vi "HTTP Error.vi"(1 "Error code options":T3={"1xx (info)"=FALSE, "2xx (success)"=FALSE, "3xx (redirect)"=FALSE, "4xx (client error)"=TRUE, "5xx (server error)"=TRUE, "Other"=TRUE}, 5 "Header":string="HTTP/1.1 301 Moved Permanently\r\nLocation: http://www.google.com/\r\nContent-Type: text/html; charset=UTF-8\r\nDate: Thu, 22 Mar 2012 21:41:48 GMT\r\nExpires: Sat, 21 Apr 2012 21:41:48 GMT\r\nCache-Control: public, max-age=2592000\r\nServer: gws\r\nContent-Length: 219\r\nX-XSS-Protection: 1; mode=block\r\nX-Frame-Options: SAMEORIGIN", 7 "body":string, 11 "error in (no error)":errorcluster) -> (4 "HTTP response code":T2, 6 "Header (dup)":string="HTTP/1.1 301 Moved Permanently\r\nLocation: http://www.google.com/\r\nContent-Type: text/html; charset=UTF-8\r\nDate: Thu, 22 Mar 2012 21:41:48 GMT\r\nExpires: Sat, 21 Apr 2012 21:41:48 GMT\r\nCache-Control: public, max-age=2592000\r\nServer: gws\r\nContent-Length: 219\r\nX-XSS-Protection: 1; mode=block\r\nX-Frame-Options: SAMEORIGIN", 8 "body (dup)":string, 10 "Header Values":T1[](array[typedef]), 14 "Error log":string, 15 "error out":errorcluster)   [LabVIEW 2020, in "Blue Easy HTTP OpenSource.lvlib"]
doc: "Turns HTTP Response Codes into the proper warning or error.\n\nHTTP 1xx Informational - Warning\nHTTP 2xx Successful - Warning\nHTTP 3xx Redirection - Error\nHTTP 4xx Client Error - Error\nHTTP 5xx Server Error - Error"
uses:
  Blue Easy HTTP OpenSource.lvlib
  HTTP error on codes.ctl
  HTTP response code.ctl
  HTTP Header.ctl
  <vilib>/dlg_ctls.llb/Space Constant.vi
  <vilib>/Utility/error.llb/Trim Whitespace.vi
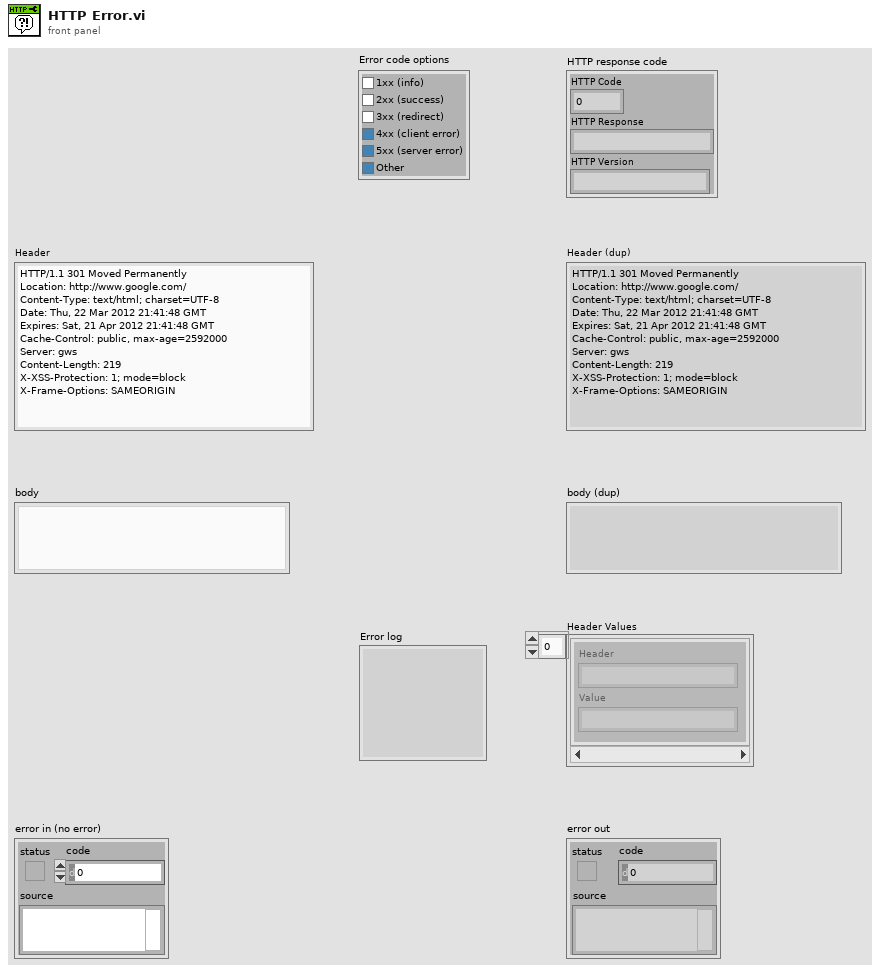
[diagram p1: front panel]
types:
  T1 = typedef "Blue Easy HTTP OpenSource.lvlib/HTTP Header.ctl" = cluster{"Header":string, "Value":string}
  T2 = typedef "Blue Easy HTTP OpenSource.lvlib/HTTP response code.ctl" = cluster{"HTTP Code":u16, "HTTP Response":string, "HTTP Version":string}
  T3 = typedef "Blue Easy HTTP OpenSource.lvlib/HTTP error on codes.ctl" = cluster{"1xx (info)":bool, "2xx (success)":bool, "3xx (redirect)":bool, "4xx (client error)":bool, "5xx (server error)":bool, "Other":bool}
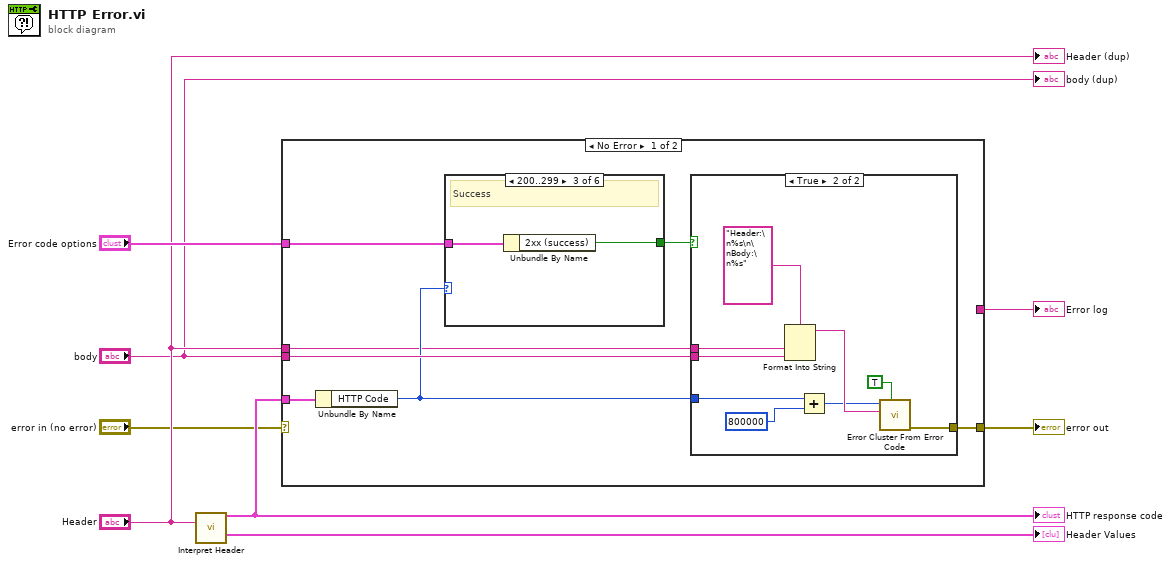
[diagram p0: block diagram]
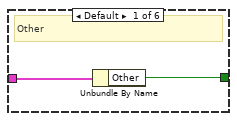
[diagram p3: hidden frame]
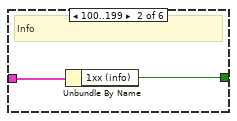
[diagram p4: hidden frame]
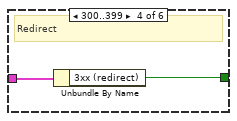
[diagram p5: hidden frame]
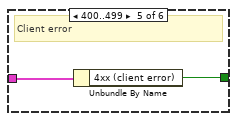
[diagram p6: hidden frame]
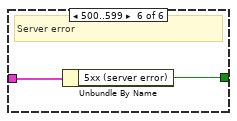
[diagram p7: hidden frame]
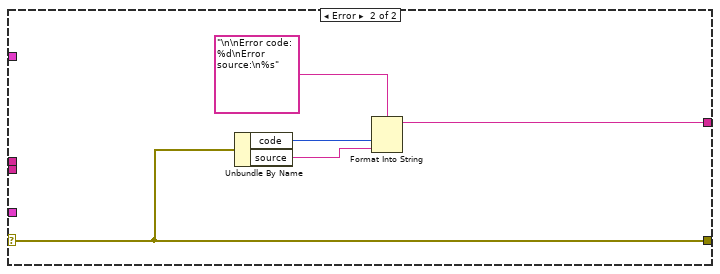
[diagram p8: hidden frame]
diagram:
  n1 = call "Interpret Header.vi"("Header"="Header") -> ("HTTP response code"=w4:T2, "Header Values"=→"Header Values":T1[])  [unwired: 11 in, 2 out]
  "HTTP response code" <- w4
  n2 = case shown="No Error" "error in (no error)" {
    selector: "error in (no error)" -> [_ w40]
    tunnel: [w15 w40] -> w8
    tunnel: "Error code options" -> [w14 _]
    tunnel: "body" -> [w12 _]
    tunnel: "Header" -> [w10 _]
    tunnel: w4 -> [w9 _]
    tunnel: [_ w37] -> w1
    frame No Error {
      n3 = Unbundle By Name(w9) -> ("HTTP Code"=w11:u16)
      n4 = case shown="200..299" w11 {
        tunnel: [w25 w27 w29 w31 w33 w35] -> w13
        tunnel: w14 -> [w26 w28 w30 w32 w34 w36]
        frame Default {
          # "Other"
          n5 = Unbundle By Name(w26) -> ("Other"=w25:bool)
        }
        frame 100..199 {
          # "Info"
          n6 = Unbundle By Name(w28) -> ("1xx (info)"=w27:bool)
        }
        frame 200..299 {
          # "Success"
          n7 = Unbundle By Name(w30) -> ("2xx (success)"=w29:bool)
        }
        frame 300..399 {
          # "Redirect"
          n8 = Unbundle By Name(w32) -> ("3xx (redirect)"=w31:bool)
        }
        frame 400..499 {
          # "Client error"
          n9 = Unbundle By Name(w34) -> ("4xx (client error)"=w33:bool)
        }
        frame 500..599 {
          # "Server error"
          n10 = Unbundle By Name(w36) -> ("5xx (server error)"=w35:bool)
        }
      }
      n11 = case shown="True" w13 {
        tunnel: [_ w24] -> w15
        tunnel: w10 -> [_ w21]
        tunnel: w12 -> [_ w20]
        tunnel: w11 -> [_ w17]
        frame False {
        }
        frame True {
          n12 = Format Into String(format string="Header:\n%s\n\nBody:\n%s", w21, w20) -> (resulting string=w19:string)  [unwired: 2 in, 1 out]
          n13 = Add(x=w17, y=800000) -> (x+y=w16:i32)
          n14 = call <vilib>:"Error Cluster From Error Code.vi"("show call chain? (False)"=TRUE, "error message (\"\")"=w19, "error code (0)"=w16) -> ("error out"=w24:errorcluster)  [unwired: 6 in]
        }
      }
    }
    frame Error {
      n15 = Unbundle By Name(w40) -> ("code"=w39:i32, "source"=w38:string)
      n16 = Format Into String(format string="\n\nError code: %d\nError source:\n%s", w39, w38) -> (resulting string=w37:string)  [unwired: 2 in, 1 out]
    }
  }
  "error out" <- w8
  "Error log" <- w1
  "Header (dup)" <- "Header"
  "body (dup)" <- "body"
